vi "Car-motor-poc.vi"() -> ()   [LabVIEW 2026]
uses:
  CTI-Grove/Examples/Sourcecode/cti-drivers-lv-visa-simple/Examples/Driver/CTIPicoVISA.lvlib
panel:
  in  "GPIO":i32=26
  in  "GPIO 2":i32=27
  in  "Duty % (0-1) 2":sgl(slide) scale=0.0..1.0
  in  "Duty % (0-1)":sgl(slide) scale=0.0..1.0
  out "Identity":T1
  in  "stop":bool
  in  "VISA resource name in":refnum<visa-resource-name>="ASRL1::INSTR"
  out "error out":errorcluster
  # "forward\n\n20 = rear left\n18 = front left\n8 = front right\n6 = rear right"
  # "https://wiki.seeedstudio.com/Grove-Passive-Buzzer/"
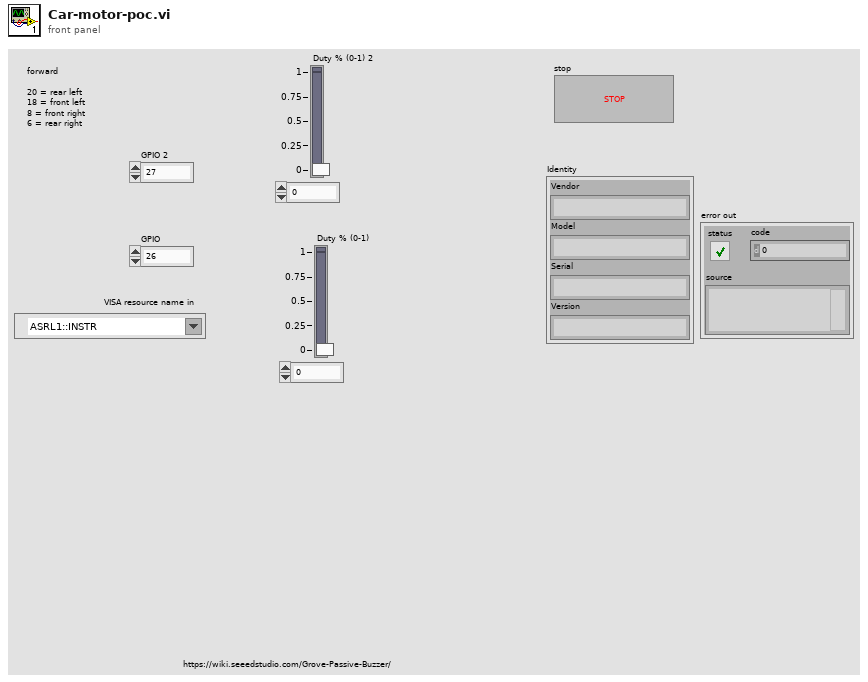
[diagram p1: front panel]
types:
  T1 = cluster{"Vendor":string, "Model":string, "Serial":string, "Version":string}
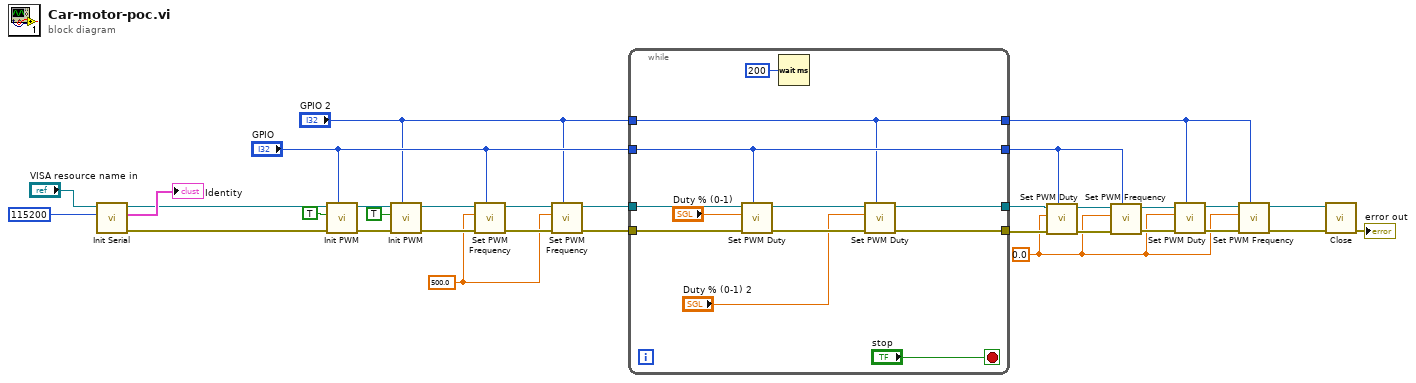
[diagram p0: block diagram]
diagram:
  w1 = sgl 500.0 ("Freq Hz")
  w10 = sgl 0.0 ("Duty % (0-1)")
  n1 = call "Init Serial.vi"("Baud (115200)"=u32 115200, "VISA resource name in"="VISA resource name in") -> ("error out"=w27:errorcluster, "Identity"=→"Identity":T1, "VISA resource name Out"=w28:refnum<visa-resource-name>)  [unwired: 7 in]
  n2 = call "Init PWM.vi"("GPIO"="GPIO", "error in (no error)"=w27, "Enable (F)"=TRUE, "VISA resource name in"=w28) -> ("error out"=w25:errorcluster, "VISA resource name"=w17:refnum<visa-resource-name>)  [unwired: 6 in]
  n3 = call "Init PWM.vi"("GPIO"="GPIO 2", "error in (no error)"=w25, "Enable (F)"=TRUE, "VISA resource name in"=w17) -> ("error out"=w18:errorcluster, "VISA resource name"=w7:refnum<visa-resource-name>)  [unwired: 6 in]
  n4 = call "Set PWM Frequency.vi"("GPIO"="GPIO", "error in (no error)"=w18, "Freq Hz"=w1, "VISA resource name in"=w7) -> ("error out"=w8:errorcluster, "VISA resource name"=w5:refnum<visa-resource-name>)  [unwired: 6 in]
  n5 = call "Set PWM Frequency.vi"("GPIO"="GPIO 2", "error in (no error)"=w8, "Freq Hz"=w1, "VISA resource name in"=w5) -> ("error out"=w6:errorcluster, "VISA resource name"=w4:refnum<visa-resource-name>)  [unwired: 6 in]
  n6 = while {
    tunnel: w4 -> [w41]
    tunnel: "GPIO" -> [w39]
    tunnel: w6 -> [w42]
    tunnel: [w37] -> w21
    tunnel: [w35] -> w22
    tunnel: [w39] -> w20
    tunnel: "GPIO 2" -> [w34]
    tunnel: [w34] -> w9
    stop <- "stop" stop-if-true
    n7 = call "Set PWM Duty.vi"("GPIO"=w39, "error in (no error)"=w42, "Duty % (0-1)"="Duty % (0-1)", "VISA resource name in"=w41) -> ("error out"=w40:errorcluster, "VISA resource name"=w36:refnum<visa-resource-name>)  [unwired: 6 in]
    n8 = Wait (ms)(milliseconds to wait=u32 200) -> ()  [unwired: 1 out]
    n9 = call "Set PWM Duty.vi"("GPIO"=w34, "error in (no error)"=w40, "Duty % (0-1)"="Duty % (0-1) 2", "VISA resource name in"=w36) -> ("error out"=w37:errorcluster, "VISA resource name"=w35:refnum<visa-resource-name>)  [unwired: 6 in]
  }
  n10 = call "Set PWM Duty.vi"("GPIO"=w20, "error in (no error)"=w21, "Duty % (0-1)"=w10, "VISA resource name in"=w22) -> ("error out"=w24:errorcluster, "VISA resource name"=w23:refnum<visa-resource-name>)  [unwired: 6 in]
  n11 = call "Set PWM Frequency.vi"("GPIO"=w20, "error in (no error)"=w24, "Freq Hz"=w10, "VISA resource name in"=w23) -> ("error out"=w19:errorcluster, "VISA resource name"=w14:refnum<visa-resource-name>)  [unwired: 6 in]
  n12 = call "Set PWM Duty.vi"("GPIO"=w9, "error in (no error)"=w19, "Duty % (0-1)"=w10, "VISA resource name in"=w14) -> ("error out"=w15:errorcluster, "VISA resource name"=w12:refnum<visa-resource-name>)  [unwired: 6 in]
  n13 = call "Set PWM Frequency.vi"("GPIO"=w9, "error in (no error)"=w15, "Freq Hz"=w10, "VISA resource name in"=w12) -> ("error out"=w13:errorcluster, "VISA resource name"=w11:refnum<visa-resource-name>)  [unwired: 6 in]
  n14 = call "Close.vi"("error in (no error)"=w13, "VISA resource name in"=w11) -> ("error out"=→"error out":errorcluster)  [unwired: 9 in]
